vi "move2Zero.vi"() -> ()   [LabVIEW 2018]
uses:
  <vilib>/Instr/_visa.llb/VISA Configure Serial Port (Instr).vi
panel:
  out "数值":dbl
  out "字符串":string
  in  "步进电机":refnum<visa-resource-name>
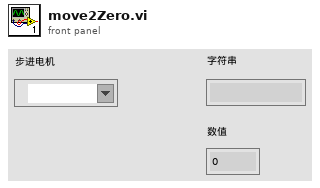
[diagram p1: front panel]
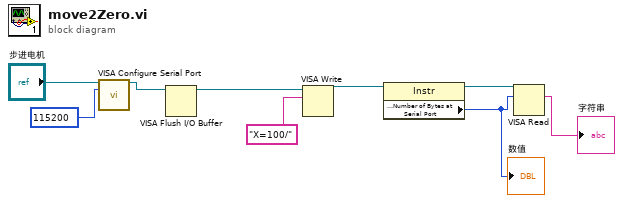
[diagram p0: block diagram]
diagram:
  n1 = call-poly "VISA Configure Serial Port"("VISA resource name"="步进电机", "baud rate (9600)"=115200) -> ("VISA resource name out"=w2:refnum<visa-resource-name>)  [unwired: 12 in, 1 out]
  n2 = VISA Flush I/O Buffer(VISA resource name=w2) -> (VISA resource name out=w1:refnum<visa-resource-name>)  [unwired: 2 in, 1 out]
  n3 = VISA Write(VISA resource name=w1, write buffer="X=100/") -> (VISA resource name out=w6:refnum<visa-resource-name>)  [unwired: 1 in, 2 out]
  n4 = property class="Instr"(reference=w6) -> (reference out=w5:refnum<visa-resource-name>, "Serial Settings:Number of Bytes at Serial Port"=w3:u32)  [unwired: 1 in, 1 out]
  "数值" <- w3
  n5 = VISA Read(VISA resource name=w5, byte count=w3) -> (read buffer=→"字符串":string)  [unwired: 1 in, 3 out]
